vi "SetLimit.vi"(7 "Low Voltage Limit (0)":dbl, 8 "error in (no error)":errorcluster, 9 "Overcurrent Protection Limit (0)":dbl, 10 "Overvoltage Protection Limit (0)":dbl, 11 "RMXPowerSupply in":refnum<class "RMX4120.lvclass">) -> (0 "error out":errorcluster, 3 "RMXPowerSupply out":refnum<class "RMX4120.lvclass">)   [LabVIEW 2023]
uses:
  Class/RMX4120_Class/RMX4120.lvclass
  D:/Projects/Repo/BTSGithubRepo/BTS5.0/ni/evo/PowerSupply/RMX412x/Support/Class/RMXPowerSupply.lvclass
  D:/Projects/Repo/BTSGithubRepo/BTS5.0/ni/evo/PowerSupply/RMX412x/Support/Class/RMX4120_Class/RMX4120.lvclass
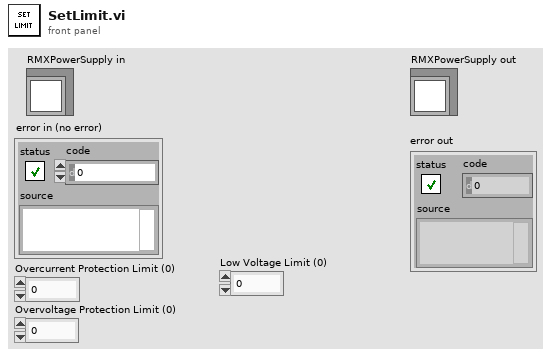
[diagram p1: front panel]
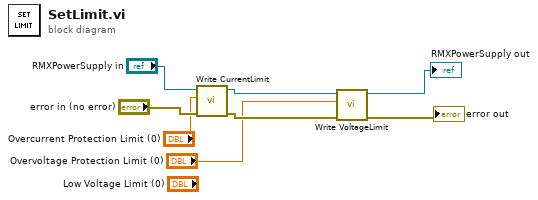
[diagram p0: block diagram]
diagram:
  n1 = call-dynamic "Write CurrentLimit.vi"("error in (no error)"="error in (no error)", "CurrentLimit"="Overcurrent Protection Limit (0)", "RMXPowerSupply in"="RMXPowerSupply in") -> ("error out"=w5:errorcluster, "RMXPowerSupply out"=w6:refnum<class "RMX4120.lvclass">)  [unwired: 7 in]
  n2 = call-dynamic "Write VoltageLimit.vi"("error in (no error)"=w5, "VoltageLimit"="Overvoltage Protection Limit (0)", "RMXPowerSupply in"=w6) -> ("error out"=→"error out":errorcluster, "RMXPowerSupply out"=→"RMXPowerSupply out":refnum<class "RMX4120.lvclass">)  [unwired: 7 in]
